vi "Simulation Configuration Read.vi"(8 "error in (no error)":errorcluster, 10 "configuration":path=path "simulation configuration.ini", 11 "simulation configuration":T1={"maxTime"=5.0, "enableVisualization"=TRUE, "Environment Definition"=path "iRobot Navigation State Machine.vi", "Record Location"=path "Simulation Record.xml", "autograde?"=TRUE, "interactive?"=FALSE, "Feedback Mode"=enum."debug navigation", "Robot State Charts"=[path "C:/Users/blueuser/Desktop/Robo Sim Berkley/cpsgrader-release-0.4/Simulators/EECS149lab/src/LabVIEW/statechart/Simulation Statechart.vi"], "statechart"=path "C:/Users/blueuser/Desktop/Robo Sim Berkley/cpsgrader-release-0.4/Simulators/EECS149lab/src/LabVIEW/statechart/Simulation Statechart.vi"}) -> (0 "error out":errorcluster, 3 "simulation configuration":T1={"maxTime"=5.0, "enableVisualization"=TRUE, "Environment Definition"=path "iRobot Navigation State Machine.vi", "Record Location"=path "Simulation Record.xml", "autograde?"=TRUE, "interactive?"=FALSE, "Feedback Mode"=enum."debug navigation", "Robot State Charts"=[path "C:/Users/blueuser/Desktop/Robo Sim Berkley/cpsgrader-release-0.4/Simulators/EECS149lab/src/LabVIEW/statechart/Simulation Statechart.vi"], "statechart"=path "C:/Users/blueuser/Desktop/Robo Sim Berkley/cpsgrader-release-0.4/Simulators/EECS149lab/src/LabVIEW/statechart/Simulation Statechart.vi"})   [LabVIEW 2015]
uses:
  CyberSim interface/Simulation Configuration.ctl
  autograder/feedbackMode.ctl
  <vilib>/Utility/config.llb/Read Key (Path).vi
  <vilib>/Utility/config.llb/Read Key (U32).vi
  <vilib>/Utility/config.llb/NI_LVConfig.lvlib
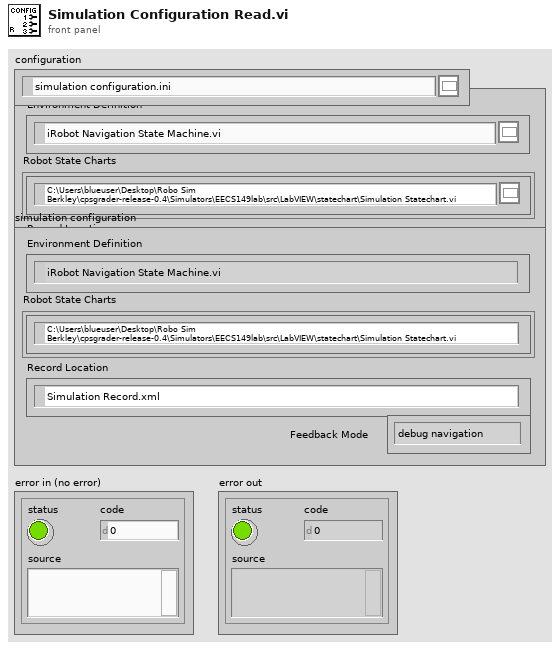
[diagram p1: front panel]
types:
  T1 = typedef "Simulation Configuration.ctl" = cluster{"maxTime":sgl, "enableVisualization":bool, "Environment Definition":path, "Record Location":path, "autograde?":bool, "interactive?":bool, "Feedback Mode":T2, "Robot State Charts":path[], "statechart":path}
  T2 = typedef "feedbackMode.ctl" = enum32{"debug navigation", "debug hill climb", "autograde navigation", "autograde hill climb"}
  T3 = typedef "NI_LVConfig.lvlib/Config Data RefNum.ctl" = refnum<k1>
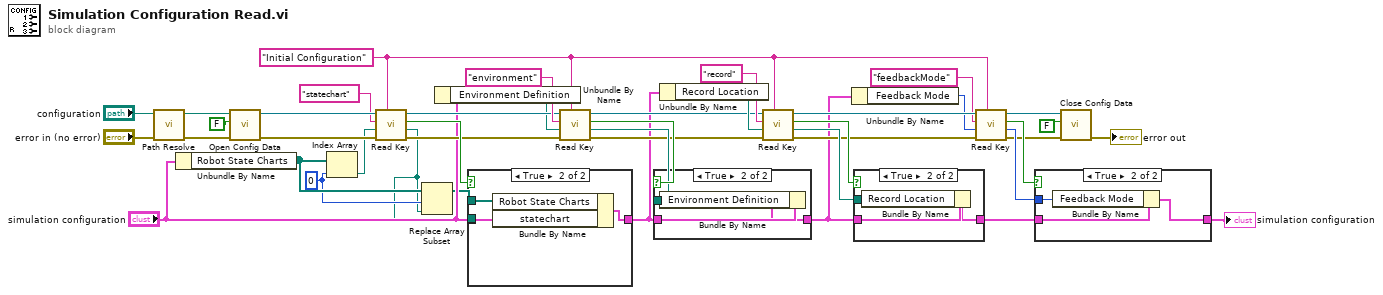
[diagram p0: block diagram]
diagram:
  w4 = 0 ("index")
  w19 = "Initial Configuration" ("section")
  n1 = call "Path Resolve.vi"("Error In"="error in (no error)", "absolute or relative path"="configuration") -> ("Error Out"=w40:errorcluster, "resolved path"=w42:path)  [unwired: 8 in]
  n2 = Unbundle By Name("simulation configuration") -> ("Robot State Charts"=w5:path[])
  n3 = call <vilib>:"Open Config Data.vi"("error in (no error)"=w40, "create file if necessary (T)"=FALSE, "configuration file path"=w42) -> ("error out"=w39:errorcluster, "refnum"=w38:T3)  [unwired: 6 in, 1 out]
  n4 = Index Array(array=w5, index=w4) -> (element=w2:path)
  n5 = call-poly <vilib>:"Read Key.vi"("section"=w19, "error in (no error)"=w39, "default value"=w2, "key"="statechart" ("string key"), "refnum"=w38) -> ("error out"=w28:errorcluster, "value"=w1:path, "found?"=w36:bool, "refnum out"=w29:T3)  [unwired: 3 in]
  n6 = Replace Array Subset(array=w5, new element=w1, index=w4) -> (w3:path[])
  n7 = Unbundle By Name("simulation configuration") -> ("Environment Definition"=w26:path)
  n8 = case shown="True" w36 {
    tunnel: "simulation configuration" -> [w43 w47]
    tunnel: [w43 w46] -> w8
    tunnel: w3 -> [_ w45]
    tunnel: w1 -> [_ w44]
    frame False {
    }
    frame True {
      n9 = Bundle By Name(cluster=w47, "Robot State Charts"=w45, "statechart"=w44) -> (w46:T1)
    }
  }
  n10 = call-poly <vilib>:"Read Key.vi"("section"=w19, "error in (no error)"=w28, "default value"=w26, "key"="environment" ("string key"), "refnum"=w29) -> ("error out"=w9:errorcluster, "value"=w34:path, "found?"=w35:bool, "refnum out"=w10:T3)  [unwired: 3 in]
  n11 = case shown="True" w35 {
    tunnel: w34 -> [_ w51]
    tunnel: w8 -> [w48 w50]
    tunnel: [w48 w49] -> w7
    frame False {
    }
    frame True {
      n12 = Bundle By Name(cluster=w50, "Environment Definition"=w51) -> (w49:T1)
    }
  }
  n13 = Unbundle By Name(w8) -> ("Record Location"=w24:path)
  n14 = call-poly <vilib>:"Read Key.vi"("section"=w19, "error in (no error)"=w9, "default value"=w24, "key"="record", "refnum"=w10) -> ("error out"=w20:errorcluster, "value"=w22:path, "found?"=w23:bool, "refnum out"=w21:T3)  [unwired: 3 in]
  n15 = Unbundle By Name(w7) -> ("Feedback Mode"=w17:T2)
  n16 = case shown="True" w23 {
    tunnel: w22 -> [_ w55]
    tunnel: w7 -> [w52 w54]
    tunnel: [w52 w53] -> w15
    frame False {
    }
    frame True {
      n17 = Bundle By Name(cluster=w54, "Record Location"=w55) -> (w53:T1)
    }
  }
  n18 = call-poly <vilib>:"Read Key.vi"("section"=w19, "error in (no error)"=w20, "default value"=w17, "key"="feedbackMode", "refnum"=w21) -> ("error out"=w11:errorcluster, "value"=w14:u32, "found?"=w16:bool, "refnum out"=w12:T3)  [unwired: 3 in]
  n19 = case shown="True" w16 {
    tunnel: w14 -> [_ w59]
    tunnel: w15 -> [w56 w58]
    tunnel: [w56 w57] -> w13
    frame False {
    }
    frame True {
      n20 = Bundle By Name(cluster=w58, "Feedback Mode"=w59) -> (w57:T1)
    }
  }
  "simulation configuration" <- w13
  n21 = call <vilib>:"Close Config Data.vi"("error in (no error)"=w11, "write file if changed (T)"=FALSE, "refnum"=w12) -> ("error out"=→"error out":errorcluster)  [unwired: 7 in, 1 out]
